vi "FlattenPageSelecter.vi"(8 "error in (no error)":errorcluster, 11 "Controls[]":refnum<vi>[](array[refnum])) -> (0 "error out":errorcluster, 3 "Flatten[]":refnum<vi>[](array[refnum]))   [LabVIEW 2019]
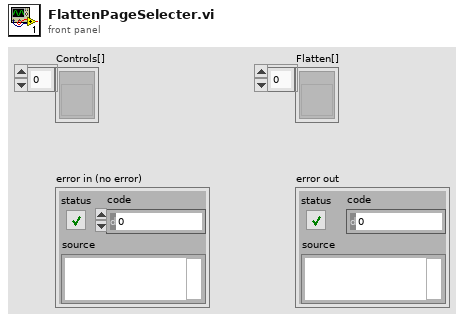
[diagram p1: front panel]
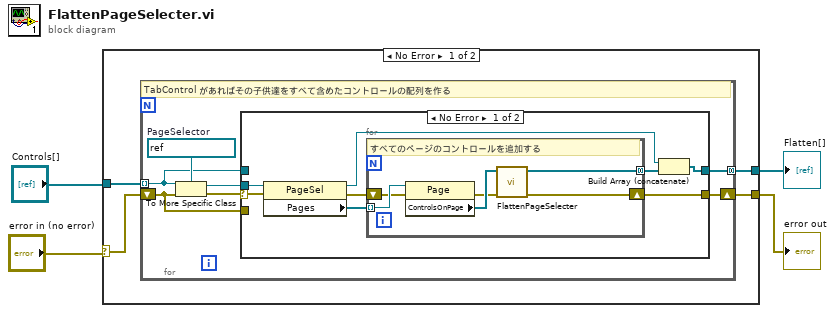
[diagram p0: block diagram]
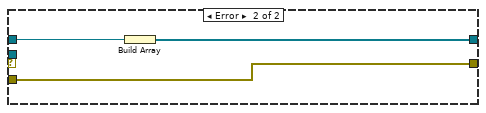
[diagram p2: hidden frame]
diagram:
  n1 = case shown="No Error" "error in (no error)" {
    selector: "error in (no error)" -> [w6 w34]
    tunnel: [w5 w33] -> w2
    tunnel: "Controls[]" -> [w8 w33]
    tunnel: [w7 w34] -> w1
    frame No Error {
      n2 = for {
        tunnel: w8 -> [w10] mode=indexing
        shift-right: [w15] -> w7
        shift-left: w6 -> [w9]
        tunnel: [w14] -> w5 mode=concatenating
        w12 = refnum<vi> refnum  # PageSelector
        # "TabControl があればその子供達をすべて含めたコントロールの配列を作る"
        n3 = To More Specific Class(target class=w12, reference=w10, error in=w9) -> (specific class reference=w13:refnum<vi>, error out=w11:errorcluster)
        n4 = case shown="No Error" w11 {
          selector: w11 -> [w18 _]
          tunnel: w13 -> [w23 _]
          tunnel: [w20 w30] -> w15
          tunnel: [w17 w31] -> w14
          tunnel: w10 -> [_ w32]
          tunnel: w9 -> [_ w30]
          frame No Error {
            n5 = property class="PageSel"(reference=w23, error in=w18) -> (reference out=w16:refnum<vi>, error out=w21:errorcluster, "Pages"=w22:refnum<vi>[])
            n6 = for {
              tunnel: w22 -> [w29] mode=indexing
              shift-right: [w25] -> w20
              shift-left: w21 -> [w28]
              tunnel: [w24] -> w19 mode=concatenating
              # "すべてのページのコントロールを追加する"
              n7 = property class="Page"(reference=w29, error in=w28) -> (error out=w26:errorcluster, "ControlsOnPage"=w27:refnum<vi>[])  [unwired: 1 out]
              n8 = call "FlattenPageSelecter.vi"("error in (no error)"=w26, "Controls[]"=w27) -> ("error out"=w25:errorcluster, "Flatten[]"=w24:refnum<vi>[])  [unwired: 8 in]
            }
            n9 = Build Array (concatenate)(w16, w19) -> (w17:refnum<vi>[])
          }
          frame Error {
            n10 = Build Array(w32) -> (w31:refnum<vi>[])
          }
        }
      }
    }
    frame Error {
    }
  }
  "Flatten[]" <- w2
  "error out" <- w1
